vi "3 - get segment values from XY data.vi"() -> ()   [LabVIEW 2013]
panel:
  in  "XY and frame data":dbl[][](array[numeric])=array14019x5[70095 elements] format="%0.3f"
  in  "appended array 2":dbl[][](array[numeric])
  in  "speed":u32(slide)
  out "Image 3":T1(plugin-control)
  in  "AVI Path":path=path "E:/PhD work/PhD research work/Videos/Chen Jin vs Hu Yun (Edited).avi"
  in  "appended array":dbl[][](array[numeric])=array1939x5[9695 elements]
  in  "Frames XY (top/bottom)":dbl[][](array[numeric])
  out "Infered action indicators":string[][](array[string])
  out "Movement data from both players":i32[][](array[numeric])
  out "Top player court segment display 2":bool[][](array[boolean])
  out "count top":i32[](graph)
  out "count bottom":i32[](graph)
  out "trans top":i32[](graph)
  out "trans bottom":i32[](graph)
  in  "ON":bool
  out "Top player court segment display":bool[][](array[boolean])
  out "Top VIew":cluster{"Numeric":dbl, "Numeric":dbl}[](graph)
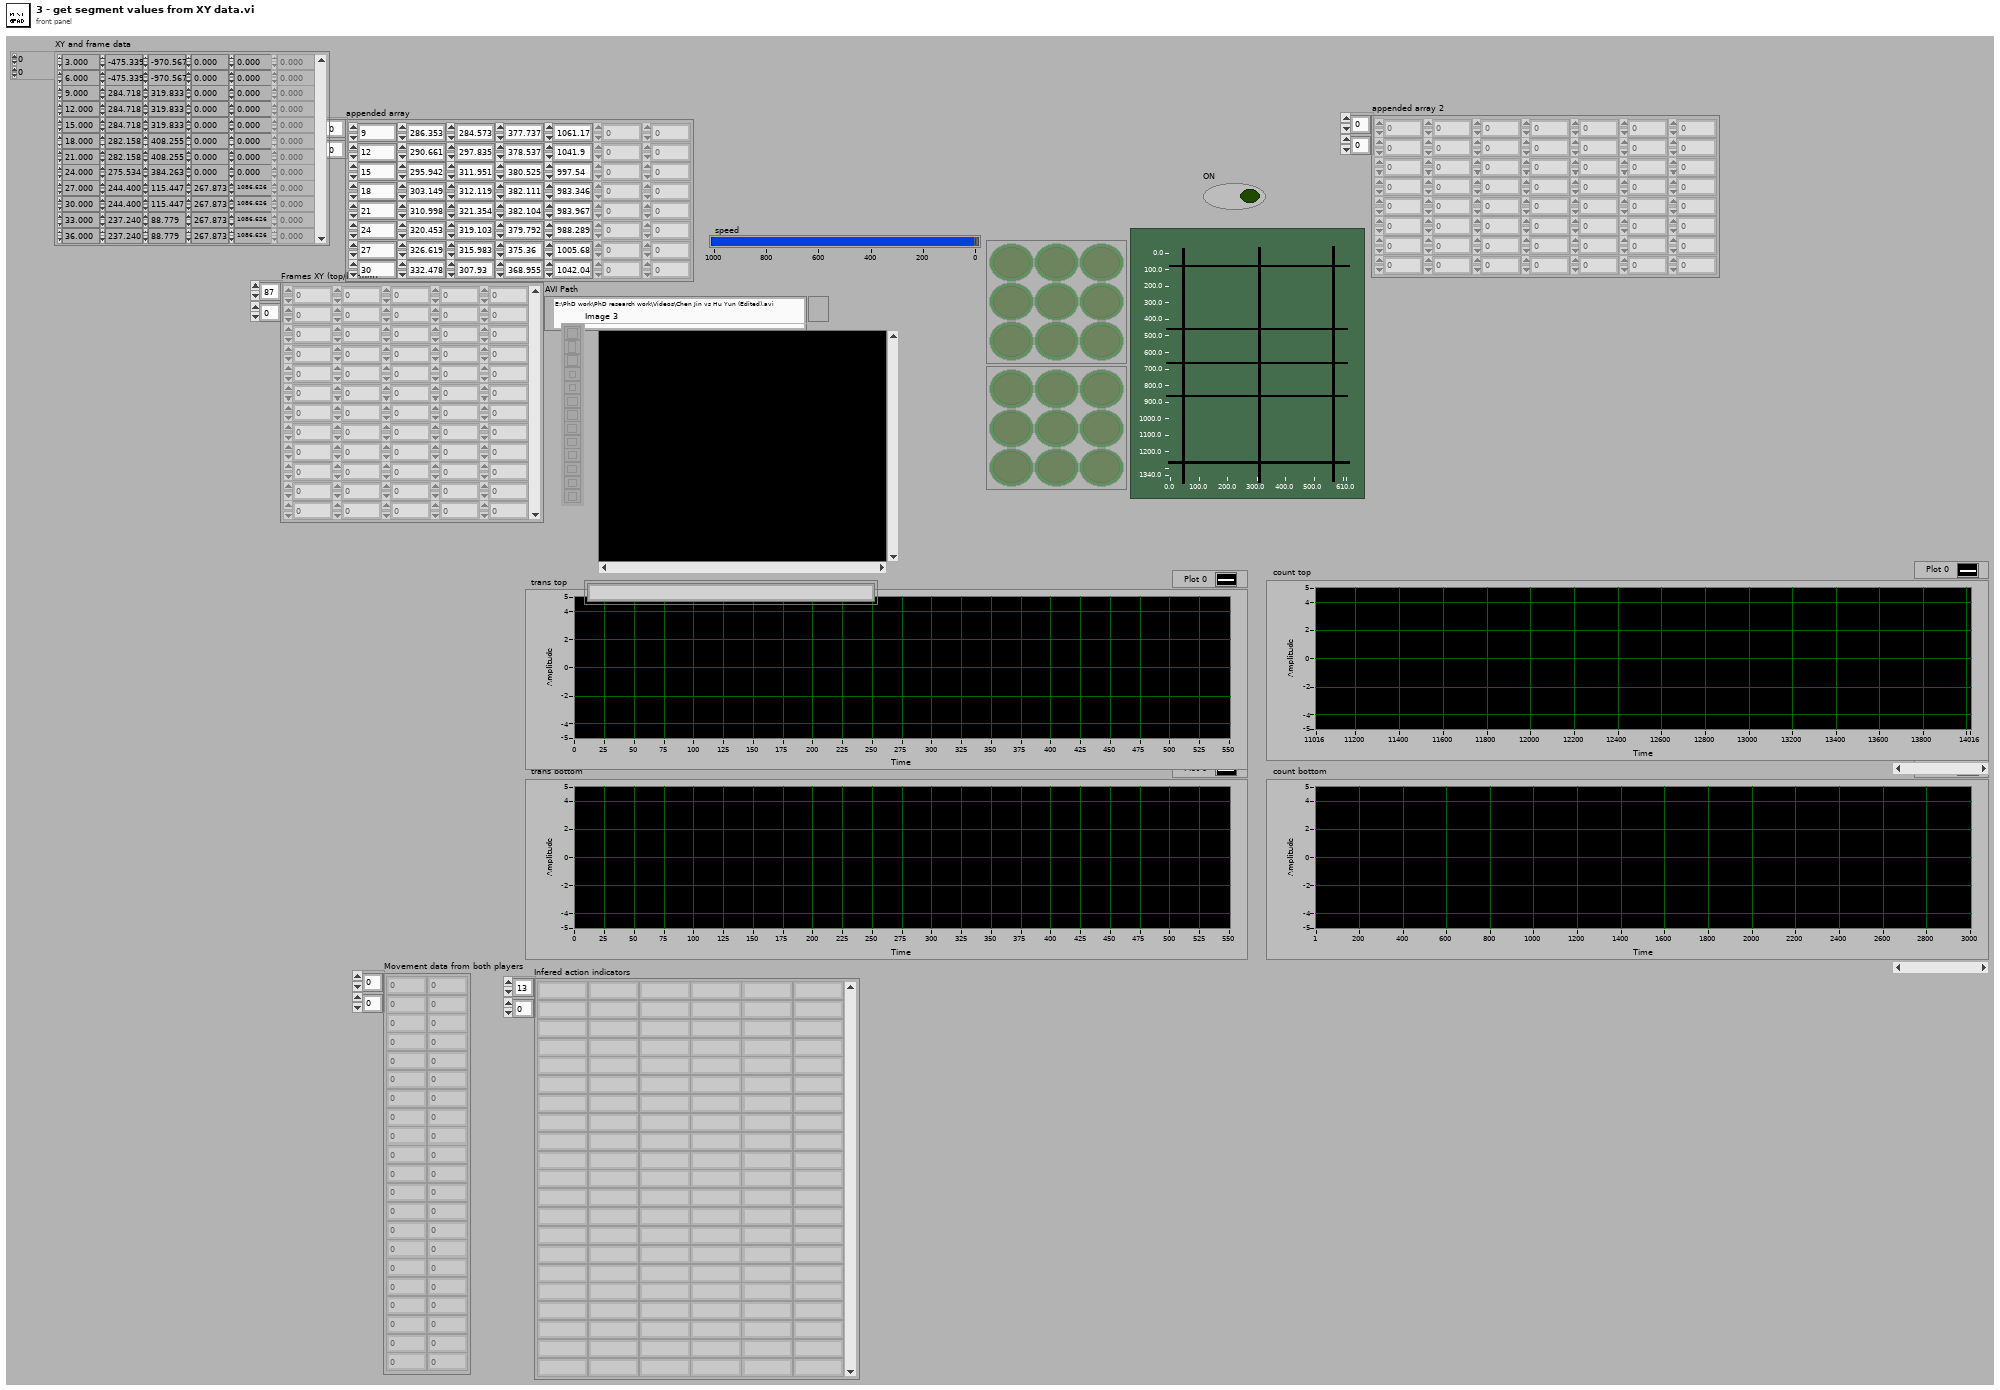
[diagram p1: front panel]
types:
  T1 = typedef "IMAQ Image.ctl" = refnum<image>
  T2 = typedef "Image Type" = u32
  T3 = typedef "AviRefnum.ctl" = refnum<k1>
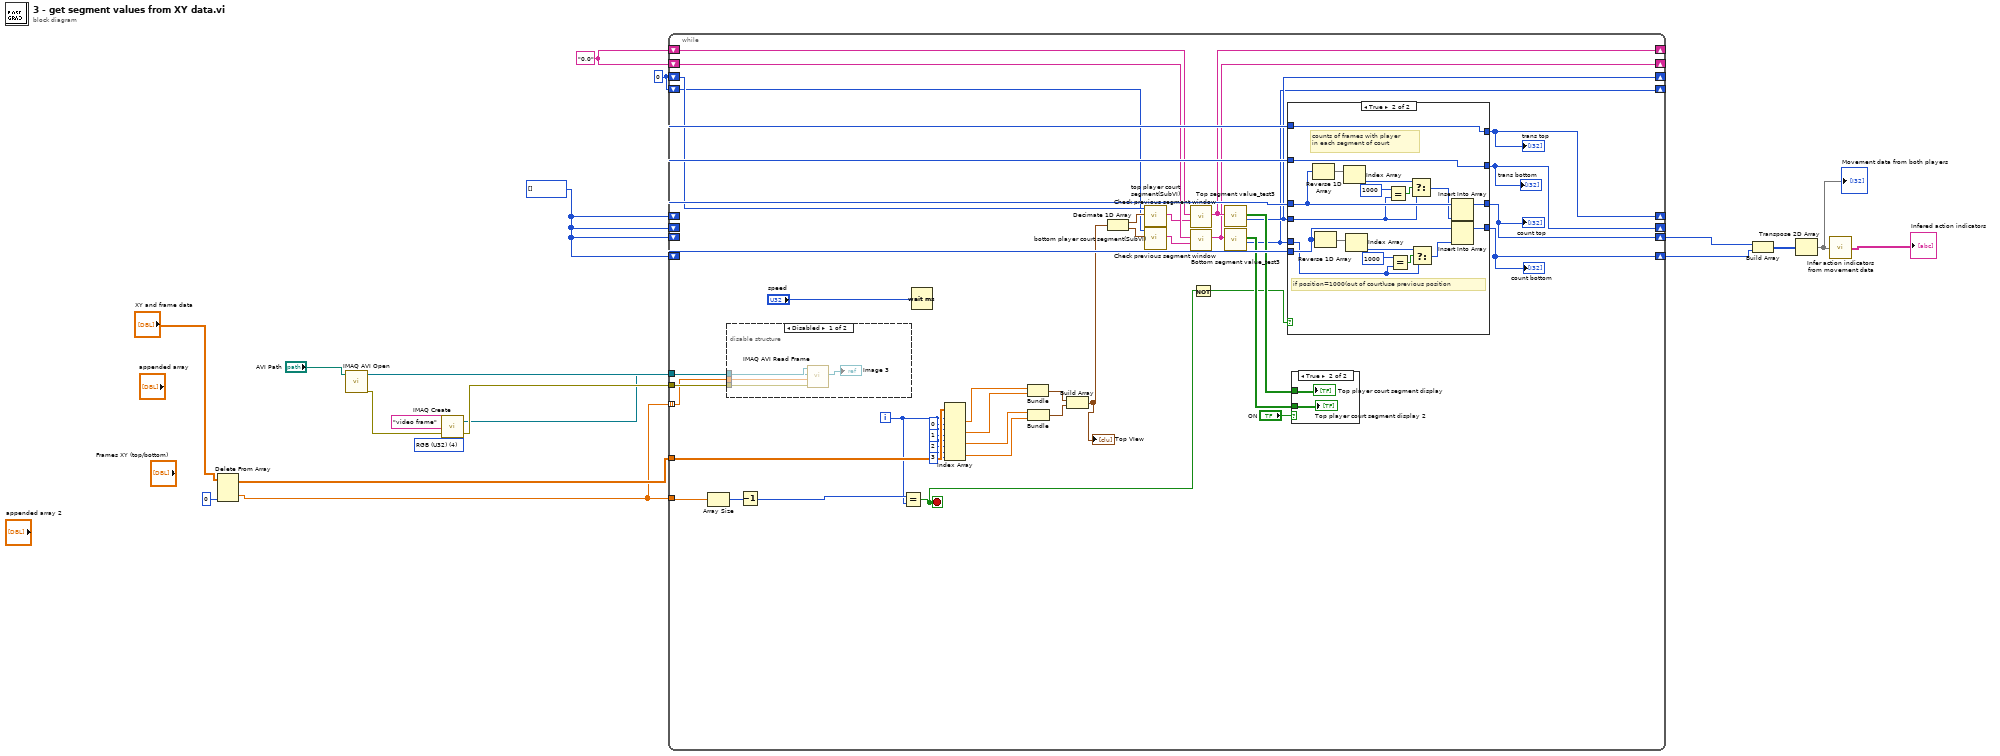
[diagram p0: block diagram]
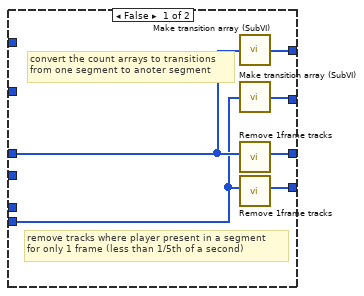
[diagram p3: hidden frame]
diagram:
  w2 = 0 ("Top player segment value")
  w8 = T2 4 items=["Grayscale (U8)", "Grayscale (I16)", "Grayscale (SGL)", "Complex (CSG)", "RGB (U32)", "HSL (U32)", "RGB (U64)", "Grayscale (U16)"] ("Image Type")
  w19 = "0,0" ("Player segment position")
  w18 = i32[] [] ("input array")
  n1 = Delete From Array(array="XY and frame data", index (col)=0 ("disabled index (col)")) -> (deleted portion=w3:dbl[], array with subset deleted=w11:dbl[][])  [unwired: 2 in]
  n2 = call "IMAQ AVI Open"("AVI Path"="AVI Path") -> ("error out"=w6:errorcluster, "Avi Refnum"=w9:T3)  [unwired: 9 in]
  n3 = call "IMAQ Create"("Image Name"="video frame", "Image Type"=w8, "error in (no error)"=w6) -> ("New Image"=w4:T1, "error out"=w5:errorcluster)  [unwired: 2 in]
  n4 = while {
    shift-right: [w45] -> w14
    shift-left: w18 -> [w60]
    shift-right: [w46] -> w13
    shift-left: w18 -> [w61]
    shift-right: [w52] -> _
    shift-left: w18 -> [w58]
    shift-right: [w57] -> _
    shift-left: w18 -> [w59]
    shift-right: [w48] -> _
    shift-left: w19 -> [w53]
    shift-right: [w49] -> _
    shift-left: w19 -> [w54]
    tunnel: w3 -> [w35]
    tunnel: w11 -> [w44]
    tunnel: w9 -> [w28]
    tunnel: w5 -> [w27]
    tunnel: w4 -> [w26]
    tunnel: w3 -> [w25] mode=indexing
    shift-right: [w23] -> _
    shift-left: w2 -> [w21]
    shift-right: [w22] -> _
    shift-left: w2 -> [w20]
    i -> [w32]
    stop <- w30 stop-if-true
    n5 = Array Size(array=w35) -> (size(s)=w34:i32)
    n6 = disable-structure shown="Disabled" {
      disable-tunnel: w28 -> [w70 _]
      disable-tunnel: w27 -> [w69 _]
      disable-tunnel: w26 -> [w68 _]
      disable-tunnel: w25 -> [w67 _]
      frame Disabled {
        n7 = call "IMAQ AVI Read Frame"("error in (no error)"=w69, "Frame Number"=w67, "Image"=w68, "Avi Refnum"=w70) -> ("Image Out"=→"Image 3":T1)  [unwired: 4 in, 3 out]
      }
      frame Enabled {
      }
    }
    n8 = Decrement(x=w34) -> (x-1=w33:i32)
    n9 = Equal?(x=w33, y=w32) -> (x = y?=w30:bool)
    n10 = Wait (ms)(milliseconds to wait="speed") -> ()  [unwired: 1 out]
    n11 = Index Array(array=w44, index (row) #1=w32, index (col) #1=0 ("disabled index (col)"), index (row) #2=w32, index (col) #2=1 ("disabled index (col)"), index (row) #3=w32, index (col) #3=2 ("disabled index (col)"), index (row) #4=w32, index (col) #4=3 ("disabled index (col)")) -> (element #1=w39:dbl, element #2=w38:dbl, element #3=w37:dbl, element #4=w36:dbl)
    n12 = Bundle(w39, w38) -> (w65:cluster{dbl, dbl})  [unwired: 1 in]
    n13 = Bundle(w37, w36) -> (w47:cluster{dbl, dbl})  [unwired: 1 in]
    n14 = Build Array(w65, w47) -> (w29:cluster{dbl, dbl}[])
    "Top VIew" <- w29
    n15 = Decimate 1D Array(w29) -> (w63:cluster{dbl, dbl}[], w64:cluster{dbl, dbl}[])
    n16 = call "top player court segment(SubVI).vi"("Top player position"=w63, "previous segment"=w21) -> ("Top player segment position"=w51:string)  [unwired: 9 in]
    n17 = call "bottom player court segment(SubVI).vi"("Bottom player position"=w64, "previous segment"=w20) -> ("Bottom player segment position"=w50:string)  [unwired: 9 in]
    n18 = call "Check previous segment window.vi"("Current player segment position"=w51, "Previous player segment position"=w54) -> ("Player segment position"=w49:string)  [unwired: 9 in]
    n19 = call "Check previous segment window.vi"("Current player segment position"=w50, "Previous player segment position"=w53) -> ("Player segment position"=w48:string)  [unwired: 9 in]
    n20 = Not(x=w30) -> (.not. x?=w31:bool)
    n21 = call "Top segment value_test3.vi"("Top player segment position"=w49) -> ("Top player segment value"=w23:i32, "Top player court segment display"=w56:bool[][])  [unwired: 9 in]
    n22 = call "Bottom segment value_test3.vi"("Bottom player segment position"=w48) -> ("Bottom player segment"=w22:i32, "Bottom player court segment display"=w55:bool[][])  [unwired: 9 in]
    n23 = case shown="True" w31 {
      tunnel: w61 -> [w74 w90]
      tunnel: w60 -> [w73 w80]
      tunnel: [w75 w91] -> w52
      tunnel: [w76 w92] -> w57
      tunnel: w22 -> [_ w77]
      tunnel: w23 -> [_ w85]
      tunnel: w59 -> [_ w92]
      tunnel: w58 -> [_ w91]
      tunnel: [w72 w94] -> w45
      tunnel: [w71 w93] -> w46
      frame False {
        # "convert the count arrays to transitions \nfrom one segment to anoter segment"
        # "remove tracks where player present in a segment \nfor only 1 frame (less than 1/5th of a second)"
        n24 = call "Make transition array (SubVI).vi"("count array in"=w74) -> ("Transition array out"=w75:i32[])
        n25 = call "Make transition array (SubVI).vi"("count array in"=w73) -> ("Transition array out"=w76:i32[])
        n26 = call "Remove 1frame tracks.vi"("count array in"=w74) -> ("count array out"=w71:i32[])  [unwired: 10 in]
        n27 = call "Remove 1frame tracks.vi"("count array in"=w73) -> ("count array out"=w72:i32[])  [unwired: 10 in]
      }
      frame True {
        # "if position=1000(out of court)use previous position"
        # "counts of frames with player\nin each segment of court"
        n28 = Reverse 1D Array(array=w90) -> (reversed array=w89:i32[])
        n29 = Reverse 1D Array(array=w80) -> (reversed array=w79:i32[])
        n30 = Index Array(array=w89) -> (element=w86:i32)  [unwired: 1 in]
        n31 = Index Array(array=w79) -> (element=w83:i32)  [unwired: 1 in]
        n32 = Equal?(x=1000 ("y"), y=w85) -> (x = y?=w87:bool)
        n33 = Equal?(x=1000 ("y"), y=w77) -> (x = y?=w82:bool)
        n34 = Select(t=w86, s=w87, f=w85) -> (s? t:f=w84:i32)
        n35 = Select(t=w83, s=w82, f=w77) -> (s? t:f=w78:i32)
        n36 = Insert Into Array(array=w90, new element=w84) -> (w93:i32[])  [unwired: 1 in]
        n37 = Insert Into Array(array=w80, new element=w78) -> (w94:i32[])  [unwired: 1 in]
      }
    }
    "trans bottom" <- w57
    "trans top" <- w52
    "count bottom" <- w45
    "count top" <- w46
    n38 = case shown="True" "ON" {
      tunnel: w56 -> [_ w96]
      tunnel: w55 -> [_ w95]
      frame False {
      }
      frame True {
        "Top player court segment display" <- w96
        "Top player court segment display 2" <- w95
      }
    }
  }
  n39 = Build Array(w13, w14) -> (w17:i32[][])
  n40 = Transpose 2D Array(2D array=w17) -> (transposed array=w15:i32[][])
  "Movement data from both players" <- w15
  n41 = call "Infer action indicators from movement data.vi"("movement data from both players"=w15) -> ("Infered action indicators"=→"Infered action indicators":string[][])
